vi "20220107_HW01_DrawCircle.vi"(1 "Offset":cluster{"X":dbl, "Y":dbl}, 2 "Radius":dbl) -> (0 "XY Graph":cluster{dbl[], dbl[]}(graph))   [LabVIEW 2019]
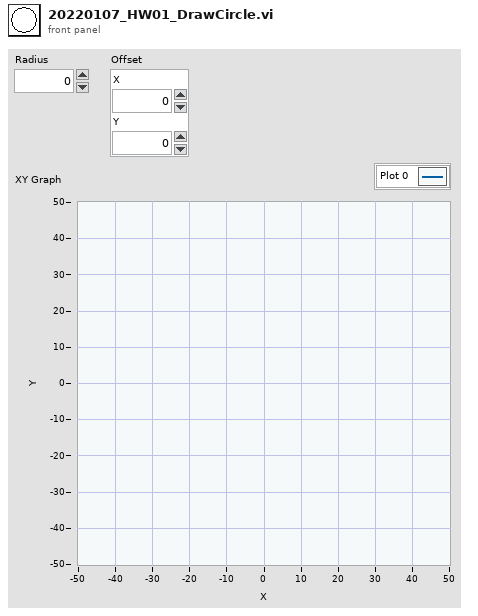
[diagram p1: front panel]
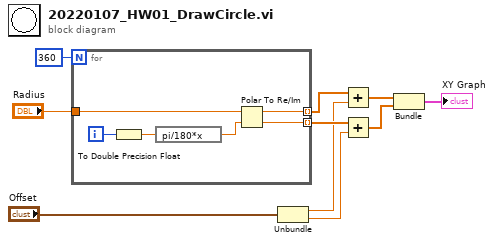
[diagram p0: block diagram]
diagram:
  n1 = for {
    N: 360 -> [_]
    tunnel: "Radius" -> [w16]
    tunnel: [w14] -> w7 mode=indexing
    tunnel: [w13] -> w6 mode=indexing
    i -> [w12]
    n2 = To Double Precision Float(number=w12) -> (double precision float=w11:dbl)
    n3 = expression code="pi/180*x"(w11) -> (w15:dbl)
    n4 = Polar To Re/Im(2:w15, 3:w16) -> (0:w13:dbl, 1:w14:dbl)
  }
  n5 = Unbundle("Offset") -> ("X"=w4:dbl, "Y"=w5:dbl)
  n6 = Add(x=w7, y=w4) -> (x+y=w3:dbl[])
  n7 = Add(x=w6, y=w5) -> (x+y=w2:dbl[])
  n8 = Bundle(w3, w2) -> (→"XY Graph":cluster{dbl[], dbl[]})  [unwired: 1 in]
